vi "jettl Msg Setup.vi"() -> (2 "Msg Strategy":refnum<class "Msg Strategy.lvclass">)   [LabVIEW 2021, in "jettl Msg Setup.lvlib"]
uses:
  jettl Msg Setup.lvlib
  jettl/Msg Strategy/Msg Strategy.lvclass
  Setup Msg Strategy/Setup Msg Strategy.lvclass
  C:/git/jettl/src/jettl/Msg Strategy/Msg Strategy.lvclass
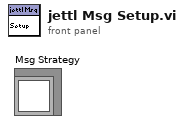
[diagram p1: front panel]
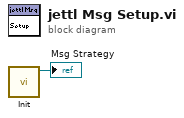
[diagram p0: block diagram]
diagram:
  n1 = call "Init.vi"() -> ("Setup Msg Strategy out"=→"Msg Strategy":refnum<class "Setup Msg Strategy.lvclass">)  [unwired: 11 in]
